vi "Add content to Engine library.vi"(6 "Project Name":string, 8 "error in (no error)":errorcluster, 9 "Project Root":path, 10 "CD Wizard - Internal Data":T1, 11 "CD Template":refnum<class "NIVS_PPL_Inline HW Interface (Inline-Async).lvclass">) -> (0 "error out":errorcluster)   [LabVIEW 2019, in "NIVS_PPL_Inline HW Interface (Inline-Async).lvclass"]
doc: "Add all virtual folders and VIs to the Engine library."
uses:
  NIVS_PPL_Inline HW Interface (Inline-Async).lvclass
  NIVS_Consolidated_CDW_MetaDataObj/Add Item - Type.ctl
  NIVS_Consolidated_CDW_MetaDataObj/NIVS_Consolidated_CDW_MetaDataObj.lvclass
  NIVS_Consolidated_CDW_MetaDataObj/CD Engine lvlib.ctl
  NIVS_Consolidated_CDW_MetaDataObj/CD Engine lvlib.vi
  NIVS_Consolidated_CDW_MetaDataObj/Internal data.ctl
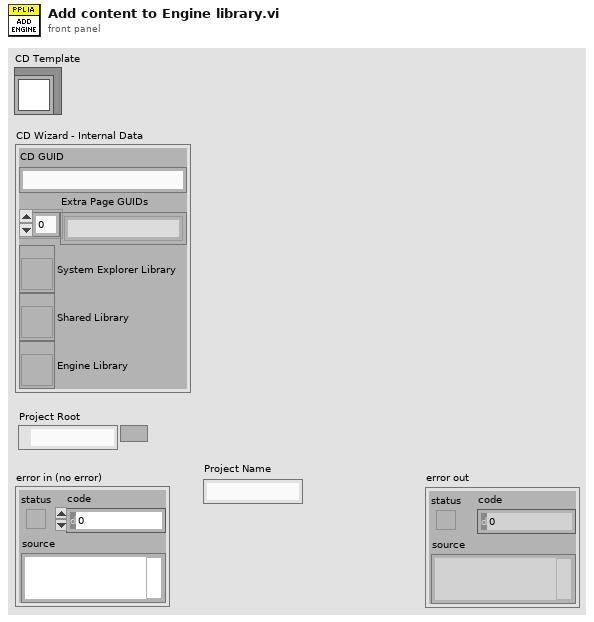
[diagram p1: front panel]
types:
  T1 = typedef "NIVS_Consolidated_CDW_MetaDataObj.lvclass/Internal data.ctl" = cluster{"CD GUID":string, "Extra Page GUIDs":string[], "System Explorer Library":refnum<vi>, "Shared Library":refnum<vi>, "Engine Library":refnum<vi>}
  T2 = typedef "NIVS_Consolidated_CDW_MetaDataObj.lvclass/CD Engine lvlib.ctl" = enum16{"LibraryFileName", "LibraryFolderName", "Engine.FolderName", "Engine.Init.FolderName", "Engine.Run.FolderName", "Engine.Shutdown.FolderName", "Types.FolderName", "Engine.RT Driver VI.TemplatePath", "Engine.RT Driver VI.FileName", "Engine.RTStateVariables.Name", "Engine.RTStateVariables.Name.NoExtension", "Engine.Async.NameExtension", "Engine.Async.TemplateName", "Engine.PPL.Async.InitVSGlobals.Name"}
  T3 = typedef "NIVS_Consolidated_CDW_MetaDataObj.lvclass/Add Item - Type.ctl" = string
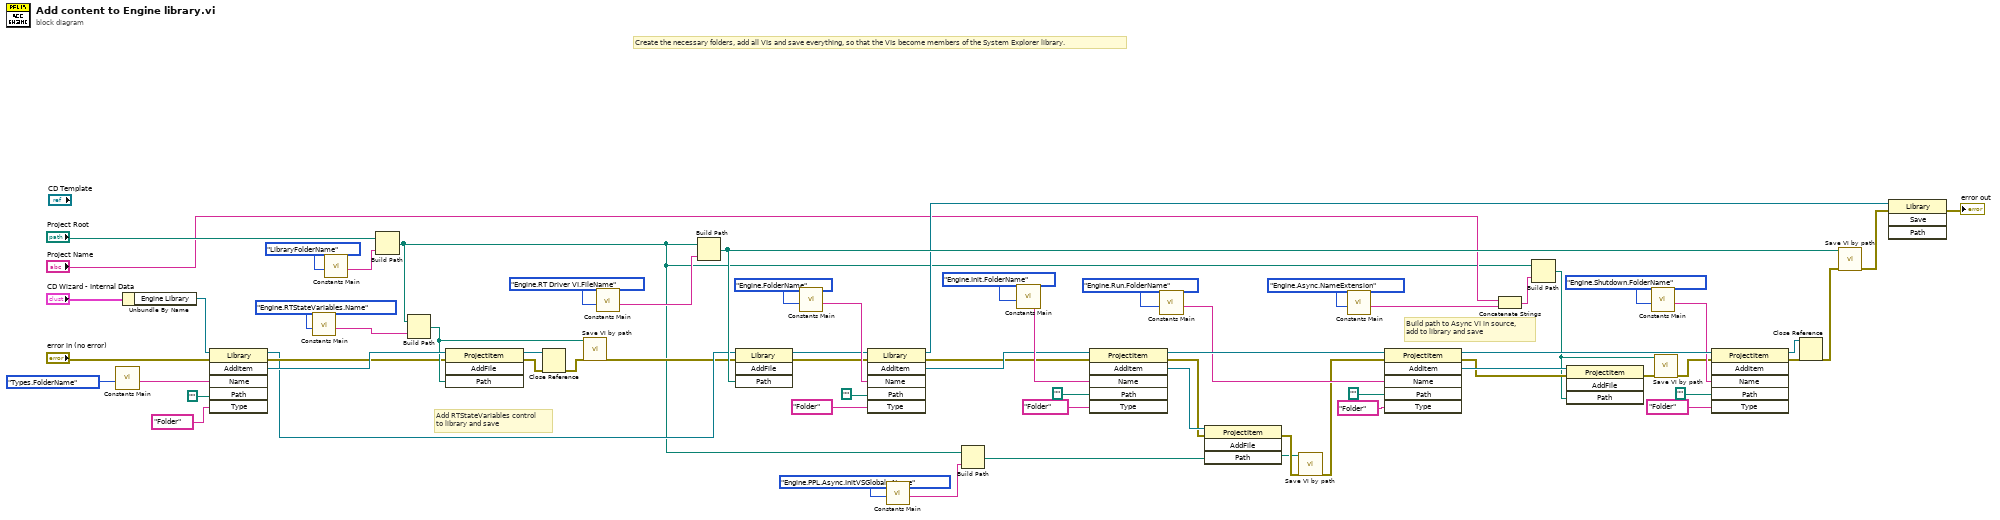
[diagram p0: block diagram]
diagram:
  # "Create the necessary folders, add all VIs and save everything, so that the VIs become members of the System Explorer library."
  # "Add RTStateVariables control\nto library and save"
  # "Build path to Async VI in source,\nadd to library and save"
  n1 = call-poly "Constants Main.vi"("Action"=CD_Engine_lvlib."Types.FolderName") -> ("Output"=w66:string)  [unwired: 10 in]
  n2 = Unbundle By Name("CD Wizard - Internal Data") -> ("Engine Library"=w56:refnum<vi>)
  n3 = invoke class="Library" method="AddItem"(reference=w56, error in="error in (no error)", "Name"=w66, "Path"=path "", "Type"=T3 "Folder" ("Add Item - Type")) -> (reference out=w20:refnum<vi>, error out=w21:errorcluster, "AddItem"=w33:refnum<vi>)  [unwired: 1 in, 3 out]
  n4 = call-poly "Constants Main.vi"("Action"=CD_Engine_lvlib."Engine.RTStateVariables.Name") -> ("Output"=w22:string)  [unwired: 10 in]
  n5 = call-poly "Constants Main.vi"("Action"=CD_Engine_lvlib."LibraryFolderName") -> ("Output"=w58:string)  [unwired: 10 in]
  n6 = Build Path(base path="Project Root", name or relative path=w58) -> (appended path=w7:path)
  n7 = Build Path(base path=w7, name or relative path=w22) -> (appended path=w31:path)
  n8 = invoke class="ProjectItem" method="AddFile"(reference=w33, error in=w21, "Path"=w31) -> (reference out=w16:refnum<vi>, error out=w32:errorcluster)  [unwired: 1 in, 2 out]
  n9 = Close Reference(reference=w16, error in (no error)=w32) -> (error out=w17:errorcluster)
  n10 = call "Save VI by path.vi"("error in (no error)"=w17, "VI path"=w31) -> ("error out"=w19:errorcluster)  [unwired: 9 in]
  n11 = call-poly "Constants Main.vi"("Action"=CD_Engine_lvlib."Engine.RT Driver VI.FileName") -> ("Output"=w60:string)  [unwired: 10 in]
  n12 = Build Path(base path=w7, name or relative path=w60) -> (appended path=w39:path)
  n13 = invoke class="Library" method="AddFile"(reference=w20, error in=w19, "Path"=w39) -> (reference out=w51:refnum<vi>, error out=w18:errorcluster)  [unwired: 1 in, 2 out]
  n14 = call-poly "Constants Main.vi"("Action"=CD_Engine_lvlib."Engine.FolderName") -> ("Output"=w53:string)  [unwired: 10 in]
  n15 = invoke class="Library" method="AddItem"(reference=w51, error in=w18, "Name"=w53, "Path"=path "", "Type"=T3 "Folder" ("Add Item - Type")) -> (reference out=w38:refnum<vi>, error out=w15:errorcluster, "AddItem"=w50:refnum<vi>)  [unwired: 1 in, 3 out]
  n16 = call-poly "Constants Main.vi"("Action"=CD_Engine_lvlib."Engine.PPL.Async.InitVSGlobals.Name") -> ("Output"=w6:string)  [unwired: 10 in]
  n17 = Build Path(base path=w7, name or relative path=w6) -> (appended path=w2:path)
  n18 = call-poly "Constants Main.vi"("Action"=CD_Engine_lvlib."Engine.Init.FolderName") -> ("Output"=w62:string)  [unwired: 10 in]
  n19 = invoke class="ProjectItem" method="AddItem"(reference=w50, error in=w15, "Name"=w62, "Path"=path "", "Type"=T3 "Folder" ("Add Item - Type")) -> (reference out=w48:refnum<vi>, error out=w4:errorcluster, "AddItem"=w5:refnum<vi>)  [unwired: 1 in, 3 out]
  n20 = call-poly "Constants Main.vi"("Action"=CD_Engine_lvlib."Engine.Run.FolderName") -> ("Output"=w46:string)  [unwired: 10 in]
  n21 = invoke class="ProjectItem" method="AddFile"(reference=w5, error in=w4, "Path"=w2) -> (error out=w3:errorcluster)  [unwired: 1 in, 3 out]
  n22 = call "Save VI by path.vi"("error in (no error)"=w3, "VI path"=w2) -> ("error out"=w1:errorcluster)  [unwired: 9 in]
  n23 = call-poly "Constants Main.vi"("Action"=CD_Engine_lvlib."Engine.Async.NameExtension") -> ("Output"=w24:string)  [unwired: 10 in]
  n24 = invoke class="ProjectItem" method="AddItem"(reference=w48, error in=w1, "Name"=w46, "Path"=path "", "Type"=T3 "Folder" ("Add Item - Type")) -> (reference out=w40:refnum<vi>, error out=w28:errorcluster, "AddItem"=w30:refnum<vi>)  [unwired: 1 in, 3 out]
  n25 = Concatenate Strings("Project Name", w24) -> (w29:string)
  n26 = Build Path(base path=w7, name or relative path=w29) -> (appended path=w26:path)
  n27 = invoke class="ProjectItem" method="AddFile"(reference=w30, error in=w28, "Path"=w26) -> (error out=w27:errorcluster)  [unwired: 1 in, 3 out]
  n28 = call-poly "Constants Main.vi"("Action"=CD_Engine_lvlib."Engine.Shutdown.FolderName") -> ("Output"=w37:string)  [unwired: 10 in]
  n29 = call "Save VI by path.vi"("error in (no error)"=w27, "VI path"=w26) -> ("error out"=w14:errorcluster)  [unwired: 9 in]
  n30 = invoke class="ProjectItem" method="AddItem"(reference=w40, error in=w14, "Name"=w37, "Path"=path "", "Type"=T3 "Folder" ("Add Item - Type")) -> (reference out=w34:refnum<vi>, error out=w36:errorcluster)  [unwired: 1 in, 4 out]
  n31 = Close Reference(reference=w34, error in (no error)=w36) -> (error out=w35:errorcluster)
  n32 = call "Save VI by path.vi"("error in (no error)"=w35, "VI path"=w39) -> ("error out"=w68:errorcluster)  [unwired: 9 in]
  n33 = invoke class="Library" method="Save"(reference=w38, error in=w68) -> (error out=→"error out":errorcluster)  [unwired: 2 in, 3 out]
